vi "Get Node Attribute (String).vi"(7 "element id":i32, 8 "error in (no error)":errorcluster, 9 "Default Value (\"\")":string, 10 "Attribute Name":string, 11 "xml":T1) -> (0 "error out":errorcluster, 1 "Attribute Value":string, 2 "found?":bool)   [LabVIEW 2011]
uses:
  Fast Parser/XML Structure - Cluster.ctl
  Fast Parser/XML Tag Type - Enum.ctl
panel:
  # "Copyright © 2006 James Kring, Inc. All rights reserved.\n\nAuthor: Jim Kring <jim.kring@jameskring.com>\n\nThis library is provided \"AS IS\" , WITHOUT WARRANTIES OR \nCONDITIONS OF ANY KIND, either express or implied.\n\nJames Kring, Inc. -- http://www.jameskring.com"
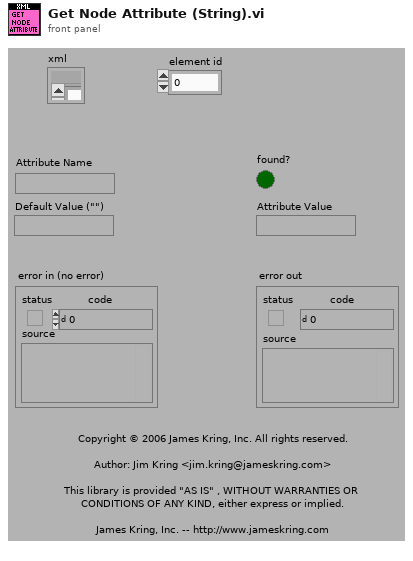
[diagram p1: front panel]
types:
  T1 = typedef "XML Structure - Cluster.ctl" = cluster{"tags":string[], "tag names":string[], "tag type":T2[], "offset":i32[], "close tag index":i32[], "xml":string, "Children":cluster{"children":i32[]}[], "parent index":i32[]}
  T2 = typedef "XML Tag Type - Enum.ctl" = enum16{"start tag", "empty tag", "end tag"}
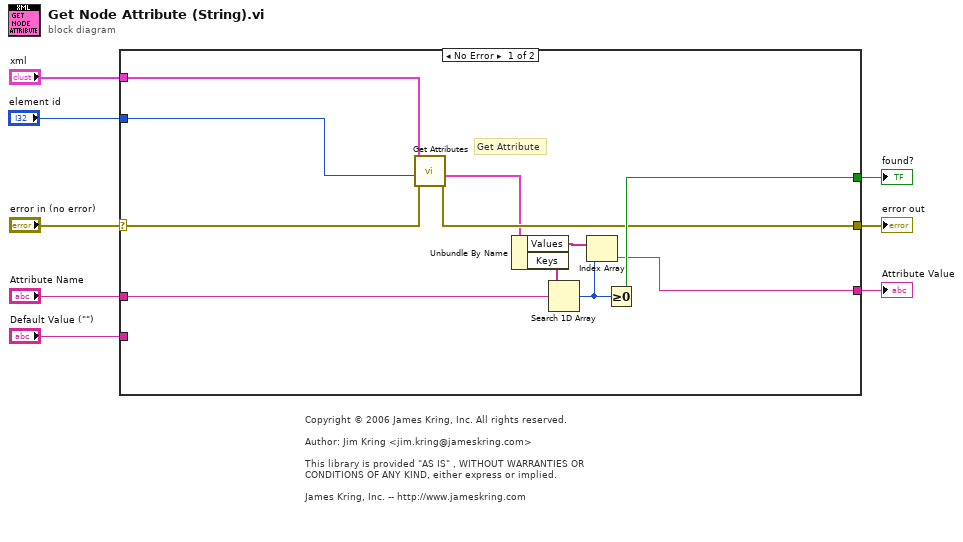
[diagram p0: block diagram]
diagram:
  # "Copyright © 2006 James Kring, Inc. All rights reserved.\n\nAuthor: Jim Kring <jim.kring@jameskring.com>\n\nThis library is provided \"AS IS\" , WITHOUT WARRANTIES OR \nCONDITIONS OF ANY KIND, either express or implied.\n\nJames Kring, Inc. -- http://www.jameskring.com"
  n1 = case shown="No Error" "error in (no error)" {
    selector: "error in (no error)" -> [w11 w20]
    tunnel: "xml" -> [w13 _]
    tunnel: [w14 _] -> w7
    tunnel: [w10 w20] -> w8
    tunnel: "Attribute Name" -> [w18 _]
    tunnel: [w17 _] -> w3
    tunnel: "Default Value (\"\")" -> [_ _]
    tunnel: "element id" -> [w12 _]
    frame No Error {
      # "Get Attribute"
      n2 = call "Get Attributes.vi"("error in (no error)"=w11, "tag index"=w12, "xml structure in"=w13) -> ("error out"=w10:errorcluster, "Attributes"=w9:cluster{"Keys":string[], "Values":string[]})  [unwired: 6 in, 1 out]
      n3 = Unbundle By Name(w9) -> ("Values"=w16:string[], "Keys"=w19:string[])
      n4 = Search 1D Array(1D array=w19, element=w18) -> (index of element=w15:i32)  [unwired: 1 in]
      n5 = Index Array(array=w16, index=w15) -> (element=w14:string)
      n6 = Greater Or Equal To 0?(x=w15) -> (x >= 0?=w17:bool)
    }
    frame Error {
    }
  }
  "error out" <- w8
  "Attribute Value" <- w7
  "found?" <- w3
